vi "GetStatus.vi"(6 "Stat Bin":refnum<vi>, 8 "error in (no error)":errorcluster, 11 "Motor in":refnum<class "Motor.lvclass">) -> (0 "error out":errorcluster, 2 "Status Int":i32, 3 "Motor out":refnum<class "Motor.lvclass">)   [LabVIEW 2012, in "Motor.lvclass"]
uses:
  Motor.lvclass
  Controlador.lvclass
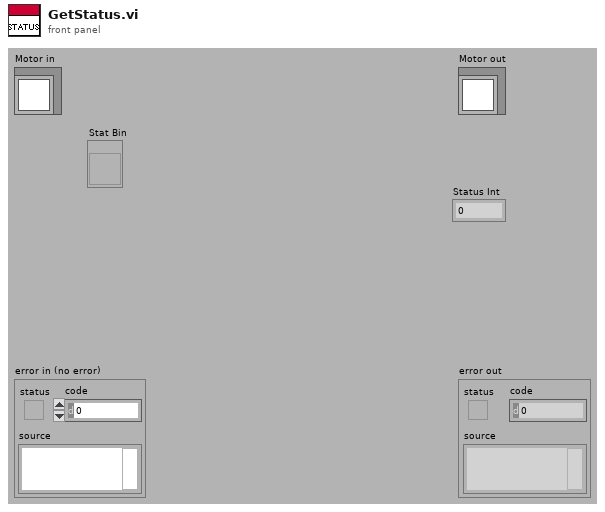
[diagram p1: front panel]
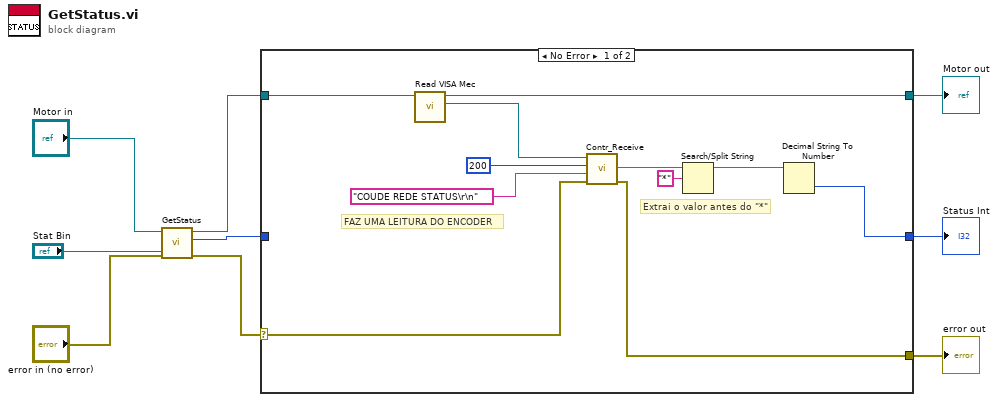
[diagram p0: block diagram]
diagram:
  n1 = call-parent "GetStatus.vi"("Stat Bin"="Stat Bin", "error in (no error)"="error in (no error)", "Device in"="Motor in") -> ("error out"=w6:errorcluster, "Status Int"=w2:i32, "Device out"=w5:refnum<class "Motor.lvclass">)  [unwired: 6 in]
  n2 = case shown="No Error" w6 {
    selector: w6 -> [w12 w22]
    tunnel: w5 -> [w14 w23]
    tunnel: [w11 w22] -> w4
    tunnel: [w13 w23] -> w3
    tunnel: w2 -> [_ w21]
    tunnel: [w10 w21] -> w1
    frame No Error {
      # "FAZ UMA LEITURA DO ENCODER"
      # "Extrai o valor antes do \"*\""
      n3 = call-dynamic "Read VISA Mec.vi"("Controlador in"=w14) -> ("VISA Mec"=w16:refnum<visa-resource-name>, "Controlador out"=w13:refnum<class "Motor.lvclass">)  [unwired: 8 in, 1 out]
      n4 = call "Contr_Receive.vi"("error in"=w12, "Command to SIFS"="COUDE REDE STATUS\r\n", "wait after tx"=u32 200, "VISA resource name"=w16) -> ("error out"=w11:errorcluster, "Response from SIFS"=w18:string)  [unwired: 2 out]
      n5 = Search/Split String(string=w18, search string/char (-)="*") -> (substring before match=w20:string)  [unwired: 1 in, 2 out]
      n6 = Decimal String To Number(string=w20) -> (number=w10:i32)  [unwired: 2 in, 1 out]
    }
    frame Error {
    }
  }
  "error out" <- w4
  "Motor out" <- w3
  "Status Int" <- w1
